vi "calculate LM.vi"() -> ()   [LabVIEW 2020]
panel:
  out "sensitivity":dbl
  in  "current level":dbl
  in  "Attenuation":dbl
  in  "current LM":dbl
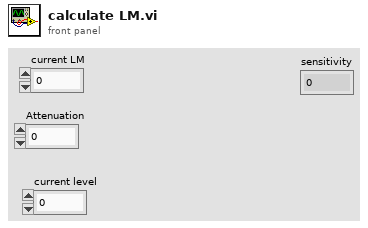
[diagram p1: front panel]
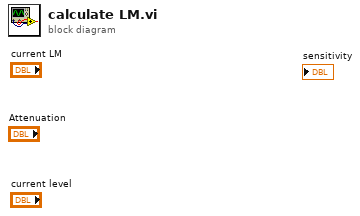
[diagram p0: block diagram]
diagram:
